vi "ScanOneChannel_DCV.vi"(7 "VISA resource name":refnum<visa-resource-name>="COM5", 8 "error in (no error)":errorcluster, 9 "Descripbe":string="Start test", 11 "Limit input":string="CH116~1.2~1.6") -> (0 "error out":errorcluster={"status"=TRUE, "code"=-1073807343, "source"="Property Node (arg 1) in VISA Configure Serial Port (Instr).vi->ReadChanel.vi->CheckTestStart.vi"}, 1 "TestData":string="0.000000-----0.000000", 2 "TestResult":bool, 3 "Limit out":string="1.2------1.6", 4 "Descripbe output":string="Start test   (CH116)", 5 "Multimeter":refnum<visa-resource-name>="USB0")   [LabVIEW 2013]
uses:
  <vilib>/Utility/error.llb/whitespace.ctl
panel:
  out "VISA resource name out":refnum<visa-resource-name>="COM5"
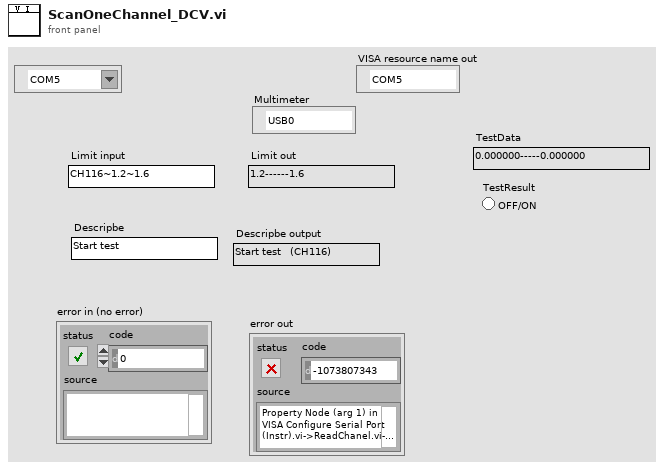
[diagram p1: front panel]
types:
  T1 = typedef "whitespace.ctl" = u16
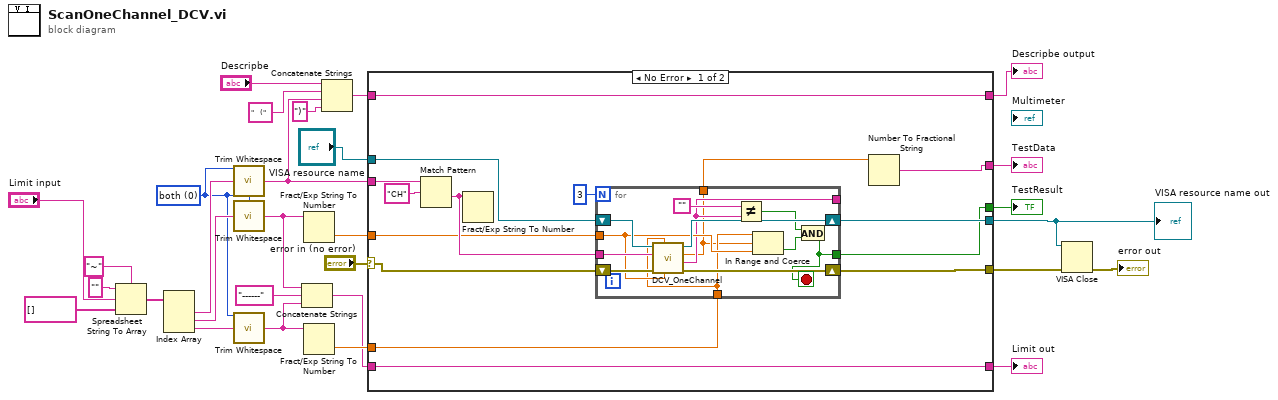
[diagram p0: block diagram]
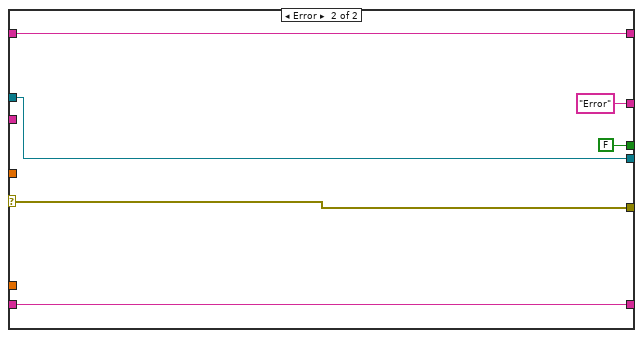
[diagram p2: hidden frame]
diagram:
  w21 = T1 0 items=["both", "start of string", "end of string"] ("location (both)")
  n1 = Spreadsheet String To Array(delimiter (Tab)="~", format string="", spreadsheet string="Limit input", array type (2D Dbl)=string[] []) -> (array=w25:string[])
  n2 = Index Array(array=w25) -> (element #1=w24:string, element #2=w23:string, element #3=w22:string)  [unwired: 3 in]
  n3 = call <vilib>:"Trim Whitespace.vi"("string"=w24, "location (both)"=w21) -> ("trimmed string"=w7:string)
  n4 = call <vilib>:"Trim Whitespace.vi"("string"=w23, "location (both)"=w21) -> ("trimmed string"=w16:string)
  n5 = call <vilib>:"Trim Whitespace.vi"("string"=w22, "location (both)"=w21) -> ("trimmed string"=w15:string)
  n6 = Concatenate Strings(w16, "------" ("string"), w15) -> (w12:string)
  n7 = Fract/Exp String To Number(string=w16) -> (number=w20:dbl)  [unwired: 3 in, 1 out]
  n8 = Fract/Exp String To Number(string=w15) -> (number=w18:dbl)  [unwired: 3 in, 1 out]
  n9 = Concatenate Strings("Descripbe", "   (" ("string"), w7, ")" ("string")) -> (w6:string)
  n10 = case shown="No Error" "error in (no error)" {
    selector: "error in (no error)" -> [w40 w63]
    tunnel: [w39 w63] -> w4
    tunnel: w7 -> [w42 _]
    tunnel: w20 -> [w34 _]
    tunnel: [w32 FALSE] -> w19
    tunnel: w18 -> [w35 _]
    tunnel: [w43 w61] -> w13
    tunnel: w12 -> [w43 w61]
    tunnel: [w41 w60] -> w11
    tunnel: w6 -> [w41 w60]
    tunnel: [w30 "Error" ("read buffer")] -> w5
    tunnel: "VISA resource name" -> [w38 w58]
    tunnel: [w37 w58] -> w1
    frame No Error {
      n11 = Match Pattern(string=w42, regular expression="CH") -> (after substring=w36:string)  [unwired: 1 in, 3 out]
      n12 = Fract/Exp String To Number(string=w36) -> ()  [unwired: 3 in, 2 out]
      n13 = for {
        N: 3 -> [_]
        tunnel: w36 -> [w53]
        shift-right: [w56] -> w39
        shift-left: w40 -> [w57]
        shift-right: [w54] -> w37
        shift-left: w38 -> [w55]
        tunnel: w35 -> [w51]
        tunnel: w34 -> [w52]
        tunnel: [w46] -> w32
        tunnel: [w49] -> _
        tunnel: [w45] -> w31
        stop <- w46 stop-if-true
        n14 = call "DCV_OneChannel.vi"("LowLimit"=w52, "HiLimit"=w51, "Error In"=w57, "Channel"=w53, "VISA resource name"=w55) -> ("Error Out"=w56:errorcluster, "Value"=w49:string, "number"=w45:dbl, "VISA resource name out"=w54:refnum<visa-resource-name>)  [unwired: 3 in]
        n15 = Not Equal?(x="", y=w49) -> (x != y?=w48:bool)
        n16 = In Range and Coerce(upper limit=w51, x=w45, lower limit=w52) -> (In Range?=w47:bool)  [unwired: 1 out]
        n17 = And(x=w48, y=w47) -> (x .and. y?=w46:bool)
      }
      n18 = Number To Fractional String(number=w31) -> (F-format string=w30:string)  [unwired: 3 in]
    }
    frame Error {
    }
  }
  "TestResult" <- w19
  "TestData" <- w5
  "Limit out" <- w13
  "Descripbe output" <- w11
  "VISA resource name out" <- w1
  n19 = VISA Close(VISA resource name=w1, error in (no error)=w4) -> (error out=→"error out":errorcluster)
